vi "Test - Navigating Structures Target.vi"() -> ()   [LabVIEW 2019]
doc: "This VI is the target for the Navigating Structures.vi example, which uses VI Scripting to determine how many case structures in this VI have constants wired to their selector terminals.\n\nDo not save changes to this VI."
panel:
  in  "Boolean":bool=TRUE
  # "Select Help>>Show Context Help and move the cursor over the VI icon to display help for this VI.\n\nDO NOT SAVE CHANGES TO THIS VI. This VI serves as the target for the Navigating Structures.vi example. Therefore, changing this VI might prevent the Navigating Structures.vi example from demonstrating its scripting task."
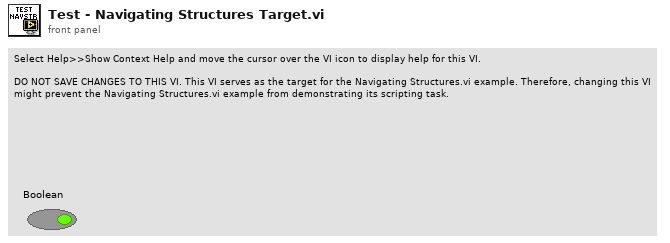
[diagram p1: front panel]
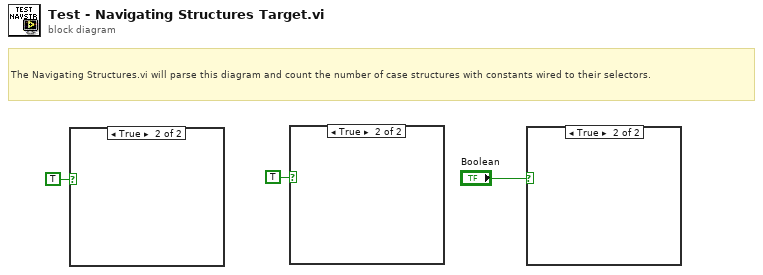
[diagram p0: block diagram]
diagram:
  # "The Navigating Structures.vi will parse this diagram and count the number of case structures with constants wired to their selectors."
  n1 = case shown="True" TRUE {
    frame False {
    }
    frame True {
    }
  }
  n2 = case shown="True" TRUE {
    frame False {
    }
    frame True {
    }
  }
  n3 = case shown="True" "Boolean" {
    frame False {
    }
    frame True {
    }
  }
